vi "createSavingCommands.vi"(1 "extension":string, 3 "Saving Path (local)":string, 4 "Save":T1) -> (0 "String":string)   [LabVIEW 2011]
uses:
  OnOffTypeDef.ctl
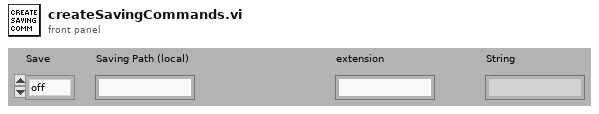
[diagram p1: front panel]
types:
  T1 = typedef "OnOffTypeDef.ctl" = enum16{"off", "on"}
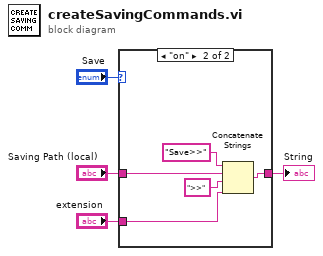
[diagram p0: block diagram]
diagram:
  n1 = case shown="\"on\"" "Save" {
    tunnel: "Saving Path (local)" -> [_ w8]
    tunnel: [_ w9] -> w3
    tunnel: "extension" -> [_ w7]
    frame "off", Default {
    }
    frame "on" {
      n2 = Concatenate Strings("Save>>" ("string"), w8, ">>" ("string"), w7) -> (w9:string)
    }
  }
  "String" <- w3
